vi "Unit Test Allow Parent Level Added False.vi"() -> ()   [LabVIEW 2019, in "Sports Unit Tests.lvclass"]
uses:
  Sports Unit Tests.lvclass
  Classes/Shaquille ONeal/Shaquille O'Neal.lvclass
  <userlib>/Blue Origin/BlueSerialization/BlueSerializer/DeserializeOptions.ctl
  <userlib>/Blue Origin/BlueSerialization/BlueSerializer/DeserializeSlicingOptions.ctl
  <userlib>/Blue Origin/BlueSerialization/BlueSerializer/DeserializeMutationOptions.ctl
  <userlib>/Blue Origin/BlueSerialization/BlueSerializer/DeserializePreservationOptions.ctl
  <userlib>/Blue Origin/BlueSerialization/BlueSerializer/PreserveNonWiredDataOption.ctl
  <vilib>/Utility/error.llb/Clear Errors.vi
  <vilib>/addons/_JKI Toolkits/Caraya/classes/Test/Define Test.vi
  <vilib>/addons/_JKI Toolkits/Caraya/classes/Assert/Assert Equal Value_Variant.vi
  <vilib>/addons/_JKI Toolkits/Caraya/classes/Assert/Assert Error.vi
  <vilib>/addons/_JKI Toolkits/Caraya/classes/Assert/Assert.lvclass
  <userlib>/Blue Origin/BlueSerialization/BlueSerializer/BlueSerializer.lvclass
panel:
  out "Table":string[][](table)=[["{\r  \"Class\":[\"Shaquille O'Neal.lvclass\",\"Sports Player.lvclass\",\"Human.lvclass\",\"BlueSerialization.lvlib:BlueSerializable.lvclass\"],\r  \"Version\":[\"2.0.0.3\",\"2.0.0.3\",\"2.0.0.3\",\"2.0.0.0\"],\r  \"BlueSerialization.lvlib:BlueSerializable.lvclass\":{\"LibVersion\":1},\r  \"Human.lvclass\":{\r    \"alive?\":true,\r    \"Age (years)\":40,\r    \"Name\":\"Shauille O'Neal\",\r    \"Height (ft)\":6\r  },\r  \"Sports Player.lvclass\":{\r    \"Professional?\":true,\r    \"Earnings (dollars)\":1000000,\r    \"Sponsor\":\"Aladin\"\r  },\r  \"Shaquille O'Neal.lvclass\":{\"#slam dunks\":768,\"Nickname\":\"Shaq\"}\r}", "{\r  \"Class\":[\"Shaquille O'Neal.lvclass\",\"Sports Player.lvclass\",\"Human.lvclass\",\"BlueSerialization.lvlib:BlueSerializable.lvclass\"],\r  \"Version\":[\"2.0.0.3\",\"2.0.0.3\",\"2.0.0.3\",\"2.0.0.0\"],\r  \"BlueSerialization.lvlib:BlueSerializable.lvclass\":{\"LibVersion\":1},\r  \"Human.lvclass\":{\r    \"alive?\":true,\r    \"Age (years)\":40,\r    \"Name\":\"Shauille O'Neal\",\r    \"Height (ft)\":6\r  },\r  \"Sports Player.lvclass\":{\r    \"Professional?\":true,\r    \"Earnings (dollars)\":1000000,\r    \"Sponsor\":\"Aladin\"\r  },\r  \"Shaquille O'Neal.lvclass\":{\"#slam dunks\":768,\"Nickname\":\"Shaq\"}\r}", "Status: FALSE\ncode: 0\n", "BlueJSONTextSerializer.lvlib:BlueJSONTextSerializer.lvclass"], ["Class = [\"Shaquille O'Neal.lvclass\", \"Sports Player.lvclass\", \"Human.lvclass\", \"BlueSerialization.lvlib:BlueSerializable.lvclass\"]\r\nVersion = [\"2.0.0.3\", \"2.0.0.3\", \"2.0.0.3\", \"2.0.0.0\"]\r\n\n[\"BlueSerialization.lvlib:BlueSerializable.lvclass\"]\nLibVersion = 1\r\n\n[\"Human.lvclass\"]\n\"alive?\" = true\r\n\"Age (years)\" = 40\r\nName = \"Shauille O'Neal\"\r\n\"Height (ft)\" = 6.0\r\n\n[\"Sports Player.lvclass\"]\n\"Professional?\" = true\r\n\"Earnings (dollars)\" = 1000000.0\r\nSponsor = \"Aladin\"\r\n\n[\"Shaquille O'Neal.lvclass\"]\n\"#slam dunks\" = 768\r\nNickname = \"Shaq\"\r\n", "Class = [\"Shaquille O'Neal.lvclass\", \"Sports Player.lvclass\", \"Human.lvclass\", \"BlueSerialization.lvlib:BlueSerializable.lvclass\"]\r\nVersion = [\"2.0.0.3\", \"2.0.0.3\", \"2.0.0.3\", \"2.0.0.0\"]\r\n\n[\"BlueSerialization.lvlib:BlueSerializable.lvclass\"]\nLibVersion = 1\r\n\n[\"Human.lvclass\"]\n\"alive?\" = true\r\n\"Age (years)\" = 40\r\nName = \"Shauille O'Neal\"\r\n\"Height (ft)\" = 6.0\r\n\n[\"Sports Player.lvclass\"]\n\"Professional?\" = true\r\n\"Earnings (dollars)\" = 1000000.0\r\nSponsor = \"Aladin\"\r\n\n[\"Shaquille O'Neal.lvclass\"]\n\"#slam dunks\" = 768\r\nNickname = \"Shaq\"\r\n", "Status: FALSE\ncode: 0\n", "BlueTOMLSerializer.lvlib:BlueTOMLSerializer.lvclass"]]
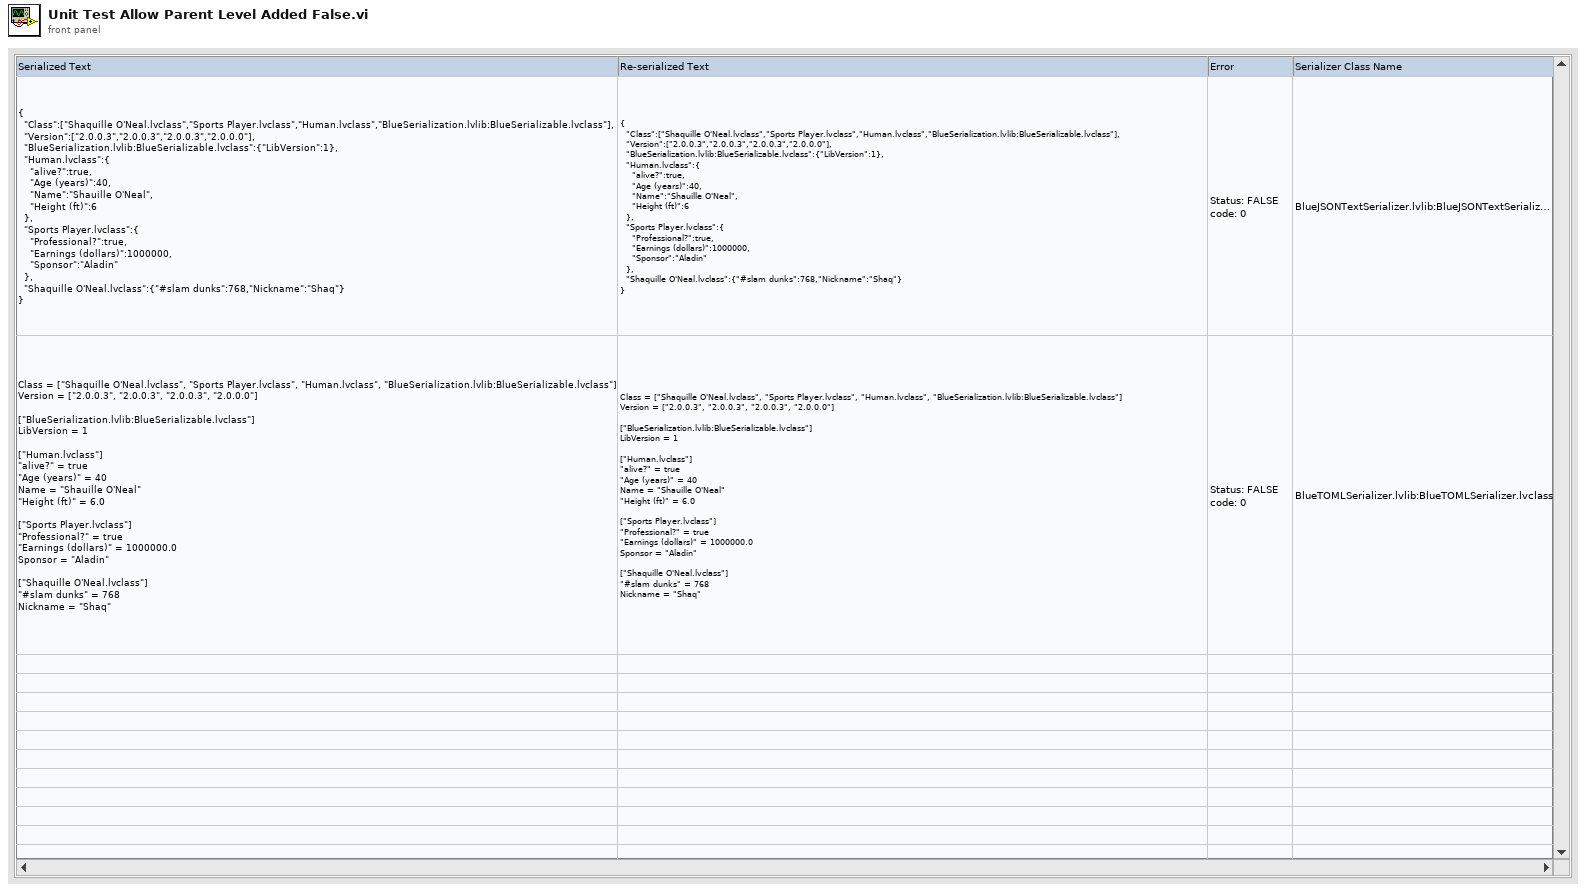
[diagram p1: front panel]
types:
  T1 = typedef "BlueSerialization.lvlib/BlueSerializer.lvclass/DeserializeOptions.ctl" = cluster{"deserialize non-BlueSerializable objects from hex?":bool, "expand objects on type conflict?":bool, "Slicing":T2, "Mutation Options":T3, "Preservation Options":T4}
  T2 = typedef "BlueSerialization.lvlib/BlueSerializer.lvclass/DeserializeSlicingOptions.ctl" = cluster{"slice flattened object data on error?":bool, "sliceable class names":string[]}
  T3 = typedef "BlueSerialization.lvlib/BlueSerializer.lvclass/DeserializeMutationOptions.ctl" = cluster{"error on inserted parent levels?":bool, "\terror on obsolete parent levels?":bool}
  T4 = typedef "BlueSerialization.lvlib/BlueSerializer.lvclass/DeserializePreservationOptions.ctl" = cluster{"Preserve wired serialized data?":bool, "Preserve wired non-serialized data":T5}
  T5 = typedef "BlueSerialization.lvlib/BlueSerializer.lvclass/PreserveNonWiredDataOption.ctl" = enum16{"Don't preserve", "Preserve (error on less-specific wired types)", "Preserve (except on less-specific wired types)"}
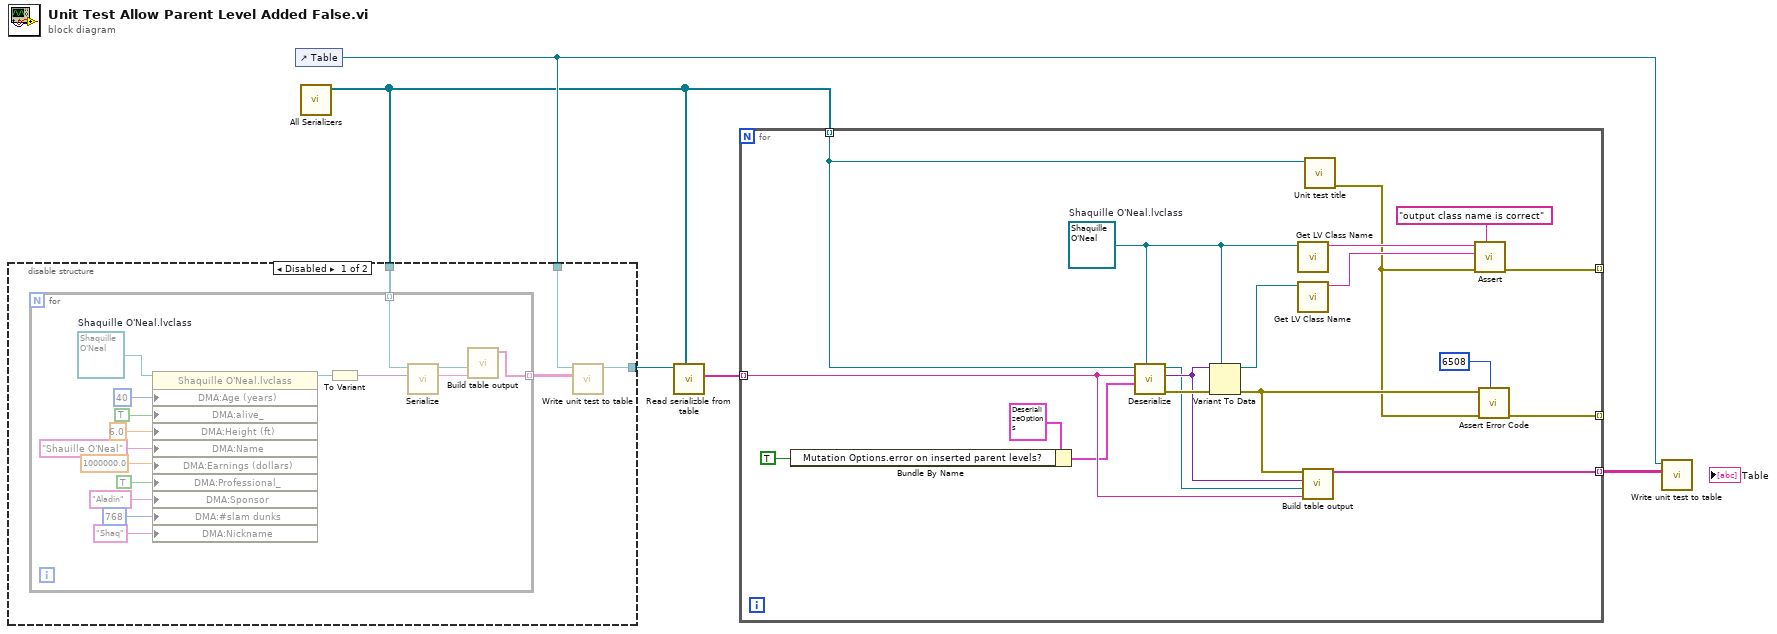
[diagram p0: block diagram]
diagram:
  n1 = control-ref of="Table"() -> (w5:refnum<vi>)
  n2 = call "All Serializers.vi"() -> ("All serializers"=w2:refnum<class "BlueSerializer.lvclass">[])  [unwired: 11 in]
  n3 = disable-structure "Diagram Disable Structure" shown="Disabled" {
    disable-tunnel: w5 -> [w8 w26]
    disable-tunnel: [w7 w26] -> w4
    disable-tunnel: w2 -> [w6 _]
    frame Disabled {
      n4 = for {
        tunnel: w6 -> [w16] mode=indexing
        tunnel: [w13] -> w9 mode=indexing
        w12 = refnum<class "Shaquille O'Neal.lvclass"> refnum  # Shaquille O'Neal.lvclass
        n5 = property on="Property Node" class="Shaquille O'Neal.lvclass"(reference=w12, "DMA:Age (years)"=u16 40 ("Age (years)"), "DMA:alive_"=TRUE ("alive_"), "DMA:Height (ft)"=6.0 ("Height (ft)"), "DMA:Name"="Shauille O'Neal" ("Name"), "DMA:Earnings (dollars)"=1000000.0 ("Earnings (dollars)"), "DMA:Professional_"=TRUE ("Professional_"), "DMA:Sponsor"="Aladin" ("Sponsor"), "DMA:#slam dunks"=u64 768 ("#slam dunks"), "DMA:Nickname"="Shaq" ("Nickname")) -> (reference out=w25:refnum<class "Shaquille O'Neal.lvclass">)  [unwired: 1 in, 1 out]
        n6 = To Variant(anything=w25) -> (Variant=w17:variant)
        n7 = call <userlib>:"Serialize.vi"("Anything"=w17, "BlueSerializer in"=w16) -> ("Serialized Text"=w15:string, "BlueSerializer out"=w14:refnum<class "BlueSerializer.lvclass">)  [unwired: 7 in, 1 out]
        n8 = call "Build table output.vi"("serialized text"=w15, "BlueSerializer in"=w14) -> ("table output"=w13:string[])  [unwired: 9 in]
      }
      n9 = call "Write unit test to table.vi"("Table"=w9, "Table ref in"=w8) -> ("Table ref out"=w7:refnum<vi>)  [unwired: 9 in]
    }
    frame Enabled {
    }
  }
  n10 = call "Read serializble from table.vi"("serializers"=w2, "Table ref in"=w4) -> ("serializable texts"=w3:string[])  [unwired: 7 in, 2 out]
  n11 = for {
    tunnel: w2 -> [w28] mode=indexing
    tunnel: [w32] -> _ mode=indexing
    tunnel: [w40] -> _ mode=indexing
    tunnel: w3 -> [w37] mode=indexing
    tunnel: [w36] -> w1 mode=indexing
    w35 = refnum<class "Shaquille O'Neal.lvclass"> refnum  # Shaquille O'Neal.lvclass
    n12 = Bundle By Name(cluster=T1 {"deserialize non-BlueSerializable objects from hex?"=FALSE, "expand objects on type conflict?"=FALSE, "Slicing"={"slice flattened object data on error?"=FALSE, "sliceable class names"=[]}, "Mutation Options"={"error on inserted parent levels?"=FALSE, "\terror on obsolete parent levels?"=FALSE}, "Preservation Options"={"Preserve wired serialized data?"=FALSE, "Preserve wired non-serialized data"=enum."Don't preserve"}} ("Deserialize Options"), "Mutation Options.error on inserted parent levels?"=TRUE ("Allow class expansion?")) -> (w27:T1)
    n13 = call <userlib>:"Deserialize.vi"("Anything"=w35, "Deserialize Options"=w27, "Serialized Text"=w37, "BlueSerializer in"=w28) -> ("error out"=w45:errorcluster, "Variant"=w39:variant, "BlueSerializer out"=w38:refnum<class "BlueSerializer.lvclass">)  [unwired: 5 in]
    n14 = Variant To Data(error in=w45, type=w35, Variant=w39) -> (data=w44:refnum<class "Shaquille O'Neal.lvclass">, error out=w34:errorcluster)
    n15 = call <vilib>:"Get LV Class Name.vi"("object"=w35) -> ("class name"=w43:string)  [unwired: 9 in, 1 out]
    n16 = call <vilib>:"Get LV Class Name.vi"("object"=w44) -> ("class name"=w42:string)  [unwired: 9 in, 1 out]
    n17 = call "Build table output.vi"("serialized text"=w37, "BlueSerializer in"=w38, "deserialized variant"=w39, "variant to data error"=w34) -> ("table output"=w36:string[])  [unwired: 7 in]
    n18 = call "Unit test title.vi"("serializer"=w28) -> ("error out"=w33:errorcluster)  [unwired: 9 in, 1 out]
    n19 = call-poly <vilib>:"Assert.vi"("Label"="output class name is correct", "error in (no error)"=w33, "Y"=w42, "X"=w43) -> ("error out"=w40:errorcluster)  [unwired: 7 in]
    n20 = call "Assert Error Code.vi"("Assert specific error code"=6508, "error in (no error)"=w33, "Error?"=w34) -> ("error out"=w32:errorcluster)  [unwired: 8 in]
  }
  n21 = call "Write unit test to table.vi"("Table"=w1, "Table ref in"=w5) -> ()  [unwired: 9 in, 1 out]
